vi "Bitstream Decode.vi"(8 "error in (no error)":errorcluster, 10 "bitstream":u8[](array[numeric]), 11 "data type":T1=enum."int") -> (0 "error out":errorcluster, 3 "Cluster":T2)   [LabVIEW 2020, in "GOLPI library.lvlib"]
uses:
  GOLPI library.lvlib
  Bitstream Data.ctl
  Bitstream Data Type.ctl
  Custom Error Codes Enum Type Def.vi
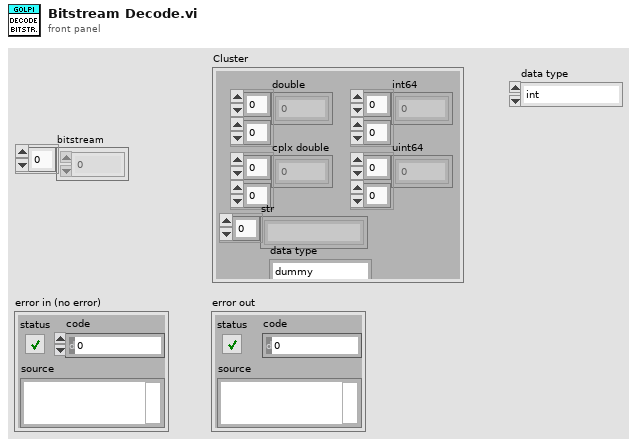
[diagram p1: front panel]
types:
  T1 = typedef "GOLPI library.lvlib/Bitstream Data Type.ctl" = enum16{"dummy", "int", "uint", "float", "complex", "str", "real numeric"}
  T2 = typedef "GOLPI library.lvlib/Bitstream Data.ctl" = cluster{"double":dbl[][], "cplx double":cdb[][], "int64":i64[][], "uint64":u64[][], "str":string[], "data type":T1}
  T3 = typedef "GOLPI library.lvlib/Custom Error Codes Enum Type Def.vi" = enum16{"no error", "00 working directory PAR1 missing", "01 octave binary PAR1 missing", "02 octave report error PAR1", "03 empty output last cmd PAR1", "04 missing temporary file PAR1", "05 pwd PAR 1 not exist", "06 oct package not installed", "07 octave default binary missing", "10 var PAR1 not string, vect", "11 var PAR1 not num, scal, ~compl", "12 var PAR1 not num, scal, compl", "13 var PAR1 not num, vect, ~compl", "14 var PAR1 not num, vect, compl", "15 var PAR1 not num, mat, ~compl", "16 var PAR1 not num, mat, ~compl", "30 read timeout", "60 bitstream transport failed", "61 bitstream decode error PAR1", "62 bitstream cannot be set", "70 struct transfer not possible", "80 struct: cluster elem. PAR1 not implem.", "81 struct: structure field PAR1 not implem.", "82 struct: size mismatch of PAR1", "83 struct: type mismatch of PAR1", "98 internal error", "99 not finished", "90 Not supported in Matlab mode", "91 Matlab variable transfer error", "92 Matlab Script Error"}
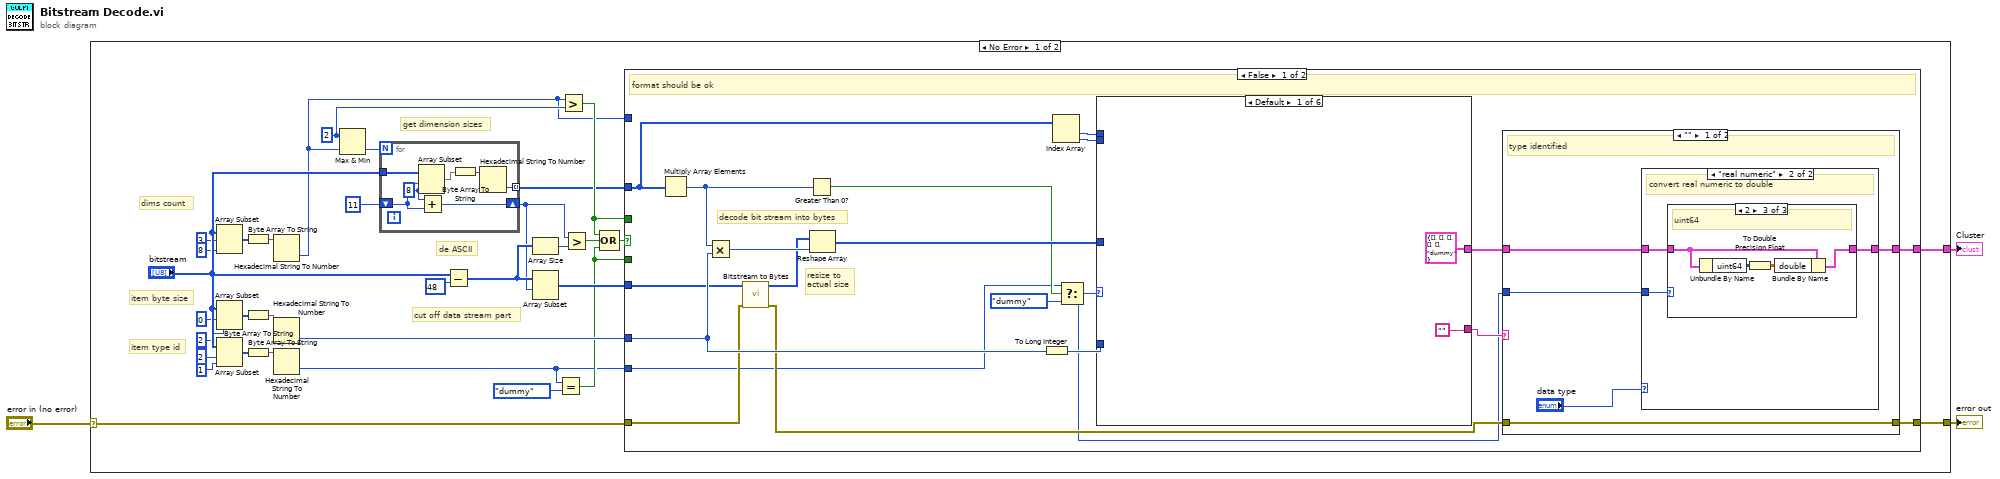
[diagram p0: block diagram]
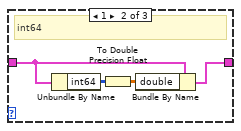
[diagram p4: hidden frame]
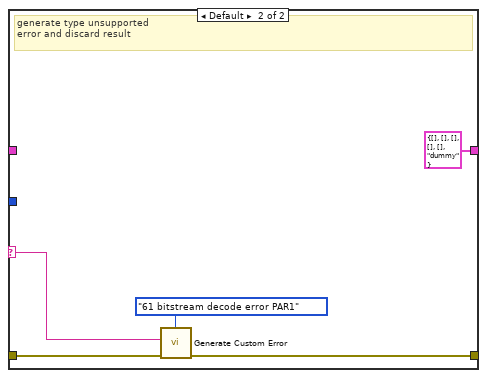
[diagram p5: hidden frame]
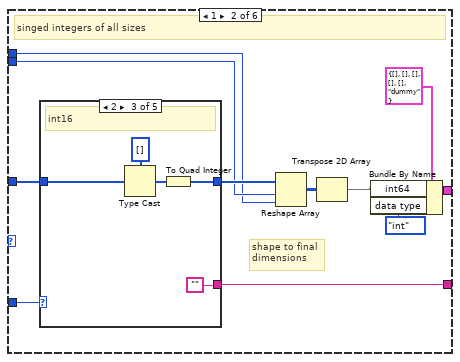
[diagram p6: hidden frame]
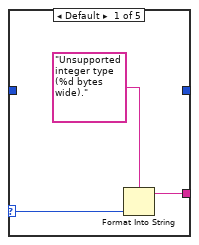
[diagram p7: hidden frame]
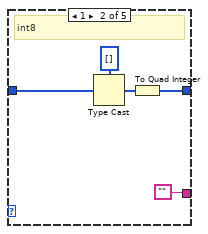
[diagram p8: hidden frame]
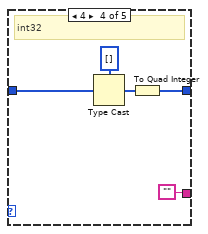
[diagram p9: hidden frame]
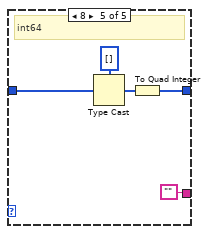
[diagram p10: hidden frame]
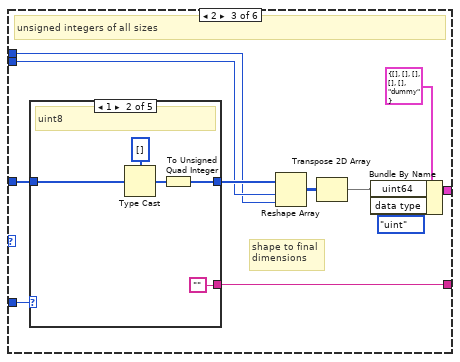
[diagram p11: hidden frame]
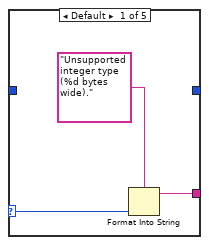
[diagram p12: hidden frame]
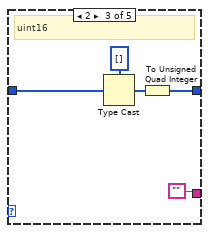
[diagram p13: hidden frame]
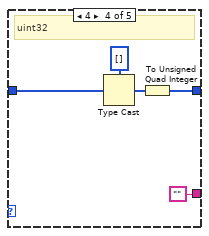
[diagram p14: hidden frame]
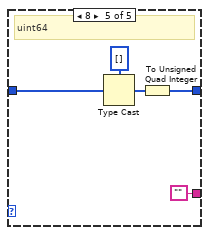
[diagram p15: hidden frame]
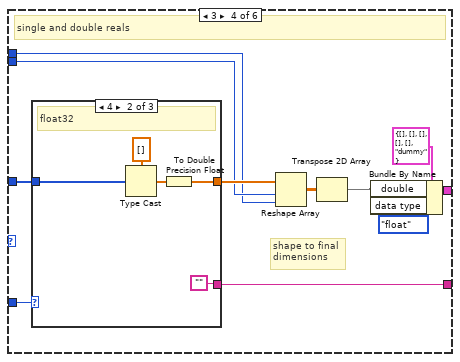
[diagram p16: hidden frame]
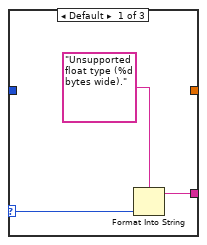
[diagram p17: hidden frame]
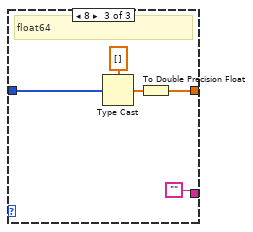
[diagram p18: hidden frame]
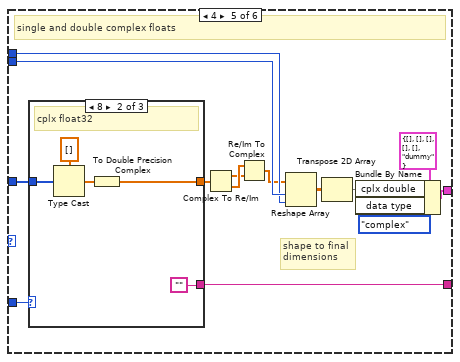
[diagram p19: hidden frame]
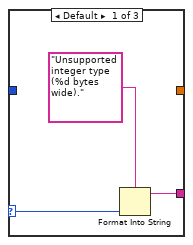
[diagram p20: hidden frame]
diagram:
  n1 = case shown="No Error" "error in (no error)" {
    selector: "error in (no error)" -> [w4 w236]
    tunnel: [w36 T2 {"double"=[], "cplx double"=[], "int64"=[], "uint64"=[], "str"=[], "data type"=enum."dummy"} ("Cluster")] -> w3
    tunnel: [w34 w236] -> w2
    frame No Error {
      w19 = u32 2 ("x")
      # "cut off data stream part"
      # "de ASCII"
      # "get dimension sizes"
      # "dims count"
      # "item type id"
      # "item byte size"
      n2 = Array Subset(array="bitstream", index=3, length=8) -> (w25:u8[])
      n3 = Array Subset(array="bitstream", index=0, length=2) -> (w32:u8[])
      n4 = Array Subset(array="bitstream", index=2, length=1) -> (w29:u8[])
      n5 = Byte Array To String(unsigned byte array=w25) -> (string=w26:string)
      n6 = Byte Array To String(unsigned byte array=w32) -> (string=w31:string)
      n7 = Byte Array To String(unsigned byte array=w29) -> (string=w30:string)
      n8 = Hexadecimal String To Number(string=w26) -> (number=w9:u32)  [unwired: 2 in, 1 out]
      n9 = Hexadecimal String To Number(string=w31) -> (number=w12:u32)  [unwired: 2 in, 1 out]
      n10 = Hexadecimal String To Number(string=w30) -> (number=w5:u32)  [unwired: 2 in, 1 out]
      n11 = Max & Min(x=w19, y=w9) -> (min(x,y)=w20:u32)  [unwired: 1 out]
      n12 = for {
        N: w20 -> [_]
        tunnel: "bitstream" -> [w234]
        shift-right: [w229] -> w17
        shift-left: 11 ("length") -> [w230]
        tunnel: [w228] -> w8 mode=indexing
        w231 = 8 ("length")
        n13 = Array Subset(array=w234, index=w230, length=w231) -> (w233:u8[])
        n14 = Add(x=w231, y=w230) -> (x+y=w229:i32)
        n15 = Byte Array To String(unsigned byte array=w233) -> (string=w232:string)
        n16 = Hexadecimal String To Number(string=w232) -> (number=w228:u32)  [unwired: 2 in, 1 out]
      }
      n17 = Subtract(x="bitstream", y=u8 48 ("length")) -> (x-y=w18:u8[])
      n18 = Array Size(array=w18) -> (size(s)=w16:i32)
      n19 = Array Subset(array=w18, index=w17) -> (w13:u8[])  [unwired: 1 in]
      n20 = Equal?(x=w5, y=Bitstream_Data_Type."dummy" ("data type")) -> (x = y?=w6:bool)
      n21 = Greater?(x=w9, y=w19) -> (0:w10:bool)
      n22 = Greater?(x=w17, y=w16) -> (0:w15:bool)
      n23 = Compound Arithmetic op=OR(w10, w15, w6) -> (w14:bool)
      n24 = case shown="False" w14 {
        tunnel: w13 -> [w45 _]
        tunnel: w8 -> [w52 _]
        tunnel: w4 -> [w42 w219]
        tunnel: [w49 w218] -> w34
        tunnel: w12 -> [w55 _]
        tunnel: [w46 T2 {"double"=[], "cplx double"=[], "int64"=[], "uint64"=[], "str"=[], "data type"=enum."dummy"} ("Cluster")] -> w36
        tunnel: w10 -> [_ w217]
        tunnel: w9 -> [_ w216]
        tunnel: w6 -> [_ w215]
        tunnel: w5 -> [w38 _]
        frame False {
          # "decode bit stream into bytes"
          # "resize to\nactual size"
          # "format should be ok"
          n25 = Multiply Array Elements(1:w52) -> (0:w41:u32)
          n26 = Multiply(x=w41, y=w55) -> (x*y=w56:u32)
          n27 = call "Bitstream to Bytes.vi"("error in (no error)"=w42, "bitstream"=w45) -> ("error out"=w43:errorcluster, "byte array"=w44:u8[])  [unwired: 8 in]
          n28 = Greater Than 0?(x=w41) -> (x > 0?=w40:bool)
          n29 = Reshape Array(w44, w56) -> (w54:u8[])
          n30 = To Long Integer(number=w55) -> (32bit integer=w53:i32)
          n31 = Index Array(array=w52) -> (element #1=w51:u32, element #2=w50:u32)  [unwired: 2 in]
          n32 = Select(t=w38, s=w40, f=Bitstream_Data_Type."dummy" ("data type")) -> (s? t:f=w37:u32)
          n33 = case shown="Default" w37 {
            tunnel: w53 -> [_ w86 w120 w154 w182 _]
            tunnel: w54 -> [_ w92 w126 w160 w187 w206]
            tunnel: w51 -> [_ w87 w121 w155 w183 w207]
            tunnel: w50 -> [_ w88 w122 w156 w184 w208]
            tunnel: [T2 {"double"=[], "cplx double"=[], "int64"=[], "uint64"=[], "str"=[], "data type"=enum."dummy"} ("Cluster") w89 w123 w157 w185 w209] -> w47
            tunnel: ["" w83 w117 w151 w175 ""] -> w48
            frame Default {
            }
            frame 1 {
              # "shape to final\ndimensions"
              # "singed integers of all sizes"
              n34 = case shown="2" w86 {
                selector: w86 -> [w94 _ _ _ _]
                tunnel: w92 -> [_ w100 w105 w110 w115]
                tunnel: [_ w97 w102 w107 w112] -> w91
                tunnel: [w93 "" "" "" ""] -> w83
                frame Default {
                  n35 = Format Into String(format string="Unsupported integer type (%d bytes wide).", w94) -> (resulting string=w93:string)  [unwired: 2 in, 1 out]
                }
                frame 1 {
                  # "int8"
                  n36 = Type Cast(type=i8[] [], x=w100) -> (*(type *) &x=w98:i8[])
                  n37 = To Quad Integer(1:w98) -> (0:w97:i64[])
                }
                frame 2 {
                  # "int16"
                  n38 = Type Cast(type=i16[] [], x=w105) -> (*(type *) &x=w103:i16[])
                  n39 = To Quad Integer(1:w103) -> (0:w102:i64[])
                }
                frame 4 {
                  # "int32"
                  n40 = Type Cast(type=i32[] [], x=w110) -> (*(type *) &x=w108:i32[])
                  n41 = To Quad Integer(1:w108) -> (0:w107:i64[])
                }
                frame 8 {
                  # "int64"
                  n42 = Type Cast(type=i64[] [], x=w115) -> (*(type *) &x=w113:i64[])
                  n43 = To Quad Integer(1:w113) -> (0:w112:i64[])
                }
              }
              n44 = Reshape Array(w91, w88, w87) -> (w85:i64[][])
              n45 = Transpose 2D Array(2D array=w85) -> (transposed array=w84:i64[][])
              n46 = Bundle By Name(cluster=T2 {"double"=[], "cplx double"=[], "int64"=[], "uint64"=[], "str"=[], "data type"=enum."dummy"} ("Cluster"), "int64"=w84, "data type"=Bitstream_Data_Type."int" ("type")) -> (w89:T2)
            }
            frame 2 {
              # "shape to final\ndimensions"
              # "unsigned integers of all sizes"
              n47 = case shown="1" w120 {
                selector: w120 -> [w128 _ _ _ _]
                tunnel: w126 -> [_ w134 w139 w144 w149]
                tunnel: [_ w131 w136 w141 w146] -> w125
                tunnel: [w127 "" "" "" ""] -> w117
                frame Default {
                  n48 = Format Into String(format string="Unsupported integer type (%d bytes wide).", w128) -> (resulting string=w127:string)  [unwired: 2 in, 1 out]
                }
                frame 1 {
                  # "uint8"
                  n49 = Type Cast(type=u8[] [], x=w134) -> (*(type *) &x=w132:u8[])
                  n50 = To Unsigned Quad Integer(1:w132) -> (0:w131:u64[])
                }
                frame 2 {
                  # "uint16"
                  n51 = Type Cast(type=u16[] [], x=w139) -> (*(type *) &x=w137:u16[])
                  n52 = To Unsigned Quad Integer(1:w137) -> (0:w136:u64[])
                }
                frame 4 {
                  # "uint32"
                  n53 = Type Cast(type=u32[] [], x=w144) -> (*(type *) &x=w142:u32[])
                  n54 = To Unsigned Quad Integer(1:w142) -> (0:w141:u64[])
                }
                frame 8 {
                  # "uint64"
                  n55 = Type Cast(type=u64[] [], x=w149) -> (*(type *) &x=w147:u64[])
                  n56 = To Unsigned Quad Integer(1:w147) -> (0:w146:u64[])
                }
              }
              n57 = Reshape Array(w125, w122, w121) -> (w119:u64[][])
              n58 = Transpose 2D Array(2D array=w119) -> (transposed array=w118:u64[][])
              n59 = Bundle By Name(cluster=T2 {"double"=[], "cplx double"=[], "int64"=[], "uint64"=[], "str"=[], "data type"=enum."dummy"} ("Cluster"), "uint64"=w118, "data type"=Bitstream_Data_Type."uint" ("type")) -> (w123:T2)
            }
            frame 3 {
              # "shape to final\ndimensions"
              # "single and double reals"
              n60 = case shown="4" w154 {
                selector: w154 -> [w162 _ _]
                tunnel: w160 -> [_ w168 w173]
                tunnel: [_ w165 w170] -> w159
                tunnel: [w161 "" ""] -> w151
                frame Default {
                  n61 = Format Into String(format string="Unsupported float type (%d bytes wide).", w162) -> (resulting string=w161:string)  [unwired: 2 in, 1 out]
                }
                frame 4 {
                  # "float32"
                  n62 = Type Cast(type=sgl[] [], x=w168) -> (*(type *) &x=w166:sgl[])
                  n63 = To Double Precision Float(number=w166) -> (double precision float=w165:dbl[])
                }
                frame 8 {
                  # "float64"
                  n64 = Type Cast(type=dbl[] [], x=w173) -> (*(type *) &x=w171:dbl[])
                  n65 = To Double Precision Float(number=w171) -> (double precision float=w170:dbl[])
                }
              }
              n66 = Reshape Array(w159, w156, w155) -> (w153:dbl[][])
              n67 = Transpose 2D Array(2D array=w153) -> (transposed array=w152:dbl[][])
              n68 = Bundle By Name(cluster=T2 {"double"=[], "cplx double"=[], "int64"=[], "uint64"=[], "str"=[], "data type"=enum."dummy"} ("Cluster"), "double"=w152, "data type"=Bitstream_Data_Type."float" ("type")) -> (w157:T2)
            }
            frame 4 {
              # "shape to final\ndimensions"
              # "single and double complex floats"
              n69 = case shown="8" w182 {
                selector: w182 -> [w189 _ _]
                tunnel: w187 -> [_ w195 w200]
                tunnel: [_ w192 w197] -> w179
                tunnel: [w188 "" ""] -> w175
                frame Default {
                  n70 = Format Into String(format string="Unsupported integer type (%d bytes wide).", w189) -> (resulting string=w188:string)  [unwired: 2 in, 1 out]
                }
                frame 8 {
                  # "cplx float32"
                  n71 = Type Cast(type=csg[] [], x=w195) -> (*(type *) &x=w193:csg[])
                  n72 = To Double Precision Complex(1:w193) -> (0:w192:cdb[])
                }
                frame 16 {
                  # "cplx float64"
                  n73 = Type Cast(type=cdb[] [], x=w200) -> (*(type *) &x=w198:cdb[])
                  n74 = To Double Precision Complex(1:w198) -> (0:w197:cdb[])
                }
              }
              n75 = Complex To Re/Im(x + iy=w179) -> (x=w177:dbl[], y=w178:dbl[])
              n76 = Re/Im To Complex(1:w177, 2:w178) -> (0:w176:cdb[])
              n77 = Reshape Array(w176, w184, w183) -> (w181:cdb[][])
              n78 = Transpose 2D Array(2D array=w181) -> (transposed array=w180:cdb[][])
              n79 = Bundle By Name(cluster=T2 {"double"=[], "cplx double"=[], "int64"=[], "uint64"=[], "str"=[], "data type"=enum."dummy"} ("Cluster"), "cplx double"=w180, "data type"=Bitstream_Data_Type."complex" ("type")) -> (w185:T2)
            }
            frame 5 {
              # "shape to final\ndimensions"
              # "string or char matrix"
              n80 = Reshape Array(w206, w208, w207) -> (w205:u8[][])
              n81 = Transpose 2D Array(2D array=w205) -> (transposed array=w204:u8[][])
              n82 = for {
                tunnel: w204 -> [w212] mode=indexing
                tunnel: [w211] -> w203 mode=indexing
                n83 = Byte Array To String(unsigned byte array=w212) -> (string=w211:string)
              }
              n84 = Bundle By Name(cluster=T2 {"double"=[], "cplx double"=[], "int64"=[], "uint64"=[], "str"=[], "data type"=enum."dummy"} ("Cluster"), "str"=w203, "data type"=Bitstream_Data_Type."str" ("type")) -> (w209:T2)
            }
          }
          n85 = case shown="\"\"" w48 {
            selector: w48 -> [_ w76]
            tunnel: w43 -> [w61 w79]
            tunnel: [w61 w78] -> w49
            tunnel: w47 -> [w60 _]
            tunnel: [w59 T2 {"double"=[], "cplx double"=[], "int64"=[], "uint64"=[], "str"=[], "data type"=enum."dummy"} ("Cluster")] -> w46
            tunnel: w37 -> [w58 _]
            frame "" {
              # "type identified"
              n86 = case shown="\"real numeric\"" "data type" {
                tunnel: w60 -> [w62 w64]
                tunnel: [w62 w63] -> w59
                tunnel: w58 -> [_ w65]
                frame Default {
                  # "strict type"
                }
                frame "real numeric" {
                  # "convert real numeric to double"
                  n87 = case shown="2" w65 {
                    tunnel: w64 -> [w66 w68 w72]
                    tunnel: [w66 w70 w74] -> w63
                    frame Default {
                    }
                    frame 1 {
                      # "int64"
                      n88 = Unbundle By Name(w68) -> ("int64"=w67:i64[][])
                      n89 = To Double Precision Float(number=w67) -> (double precision float=w69:dbl[][])
                      n90 = Bundle By Name(cluster=w68, "double"=w69) -> (w70:T2)
                    }
                    frame 2 {
                      # "uint64"
                      n91 = Unbundle By Name(w72) -> ("uint64"=w71:u64[][])
                      n92 = To Double Precision Float(number=w71) -> (double precision float=w73:dbl[][])
                      n93 = Bundle By Name(cluster=w72, "double"=w73) -> (w74:T2)
                    }
                  }
                }
              }
            }
            frame Default {
              # "generate type unsupported\nerror and discard result"
              n94 = call "Generate Custom Error.vi"("error in"=w79, "PAR1"=w76, "GOLPI error"=Custom_Error_Codes_Enum_Type_Def.vi."61 bitstream decode error PAR1") -> ("error out"=w78:errorcluster)  [unwired: 8 in]
            }
          }
        }
        frame True {
          # "bitstream is not ok"
          n95 = case shown="False" w217 {
            tunnel: w216 -> [w223 _]
            tunnel: [w222 w225] -> w214
            tunnel: w215 -> [_ w224]
            frame True {
              n96 = Format Into String(format string="Variable dimensions mismatch! Object dimensions count (%d) can't be higher than 2.", w223) -> (resulting string=w222:string)  [unwired: 2 in, 1 out]
            }
            frame False {
              n97 = case shown="True" w224 {
                tunnel: ["Variable type or dimensions doesn't match required type!" ("format string") "Stream seems to be incomplete! Possibly timeout reached." ("format string")] -> w225
                frame True {
                }
                frame False {
                }
              }
            }
          }
          n98 = call "Generate Custom Error.vi"("error in"=w219, "PAR1"=w214, "GOLPI error"=Custom_Error_Codes_Enum_Type_Def.vi."61 bitstream decode error PAR1") -> ("error out"=w218:errorcluster)  [unwired: 8 in]
        }
      }
    }
    frame Error {
    }
  }
  "Cluster" <- w3
  "error out" <- w2
